vi "Set Valve Status.vi"(7 "Valve Status":T1, 8 "error in (no error)":errorcluster, 11 "Aalborg GFC17 in":refnum<class "Aalborg GFC17.lvclass">) -> (0 "error out":errorcluster, 3 "Aalborg GFC17 out":refnum<class "Aalborg GFC17.lvclass">)   [LabVIEW 2011, in "Aalborg GFC17.lvclass"]
uses:
  Aalborg GFC17.lvclass
  Mass Flow Controller/Valve Status.ctl
  Aalborg GFC17.lvclass/Aalborg GFC17.ctl
  <vilib>/DAQmx/write.llb/DAQmx Write (Analog DBL 1Chan 1Samp).vi
  <vilib>/DAQmx/miscellaneous.llb/DAQmx Fill In Error Info.vi
  Mass Flow Controller/Mass Flow Controller.lvclass
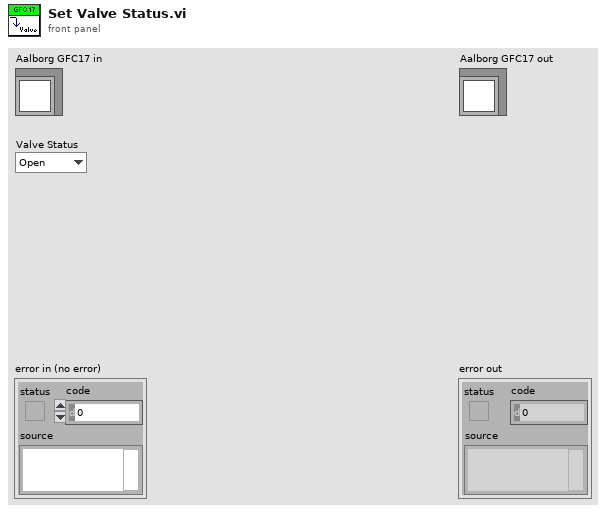
[diagram p1: front panel]
types:
  T1 = typedef "Mass Flow Controller.lvclass/Valve Status.ctl" = enum16{"Open", "Closed"}
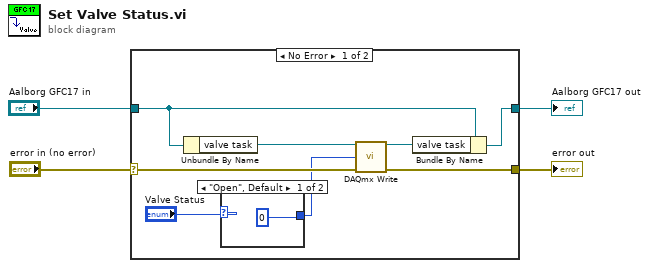
[diagram p0: block diagram]
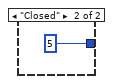
[diagram p2: hidden frame]
diagram:
  n1 = case shown="No Error" "error in (no error)" {
    selector: "error in (no error)" -> [w11 w16]
    tunnel: [w7 w16] -> w3
    tunnel: [w8 w15] -> w1
    tunnel: "Aalborg GFC17 in" -> [w10 w15]
    frame No Error {
      n2 = Unbundle By Name(w10) -> ("valve task"=w12:refnum<k21>)
      n3 = case shown="\"Open\", Default" "Valve Status" {
        tunnel: [0 5] -> w5
        frame "Open", Default {
        }
        frame "Closed" {
        }
      }
      n4 = call-poly <vilib>:"DAQmx Write.vi"("task/channels in"=w12, "data"=w5, "error in"=w11) -> ("task out"=w9:refnum<k21>, "error out"=w7:errorcluster)  [unwired: 10 in, 1 out]
      n5 = Bundle By Name(cluster=w10, "valve task"=w9) -> (w8:refnum<class "Aalborg GFC17.lvclass">)
    }
    frame Error {
    }
  }
  "error out" <- w3
  "Aalborg GFC17 out" <- w1
